vi "niRFSysCalReader Close.vi"(8 "error in":errorcluster, 11 "niRFSysCalReader Handle":T1) -> (0 "error out":errorcluster)   [LabVIEW 2016, in "niRFSysCalReader.lvlib"]
doc: "Releases the application memory created by the <b>niRFSysCalReader Initialize.vi</b>"
uses:
  niRFSysCalReader.lvlib
  _INCLUDES/niRFSysCalReader Handle.ctl
  _INCLUDES/niRFSysCalReader Core States.ctl
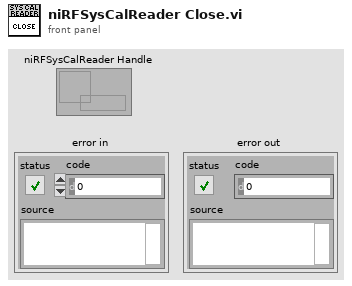
[diagram p1: front panel]
types:
  T1 = typedef "niRFSysCalReader.lvlib/niRFSysCalReader Handle.ctl" = refnum<data-value>
  T2 = typedef "niRFSysCalReader.lvlib/niRFSysCalReader Core States.ctl" = enum16{"Initialize", "Interpolator State", "Add Pathloss", "Get Pathloss", "Remove Pathloss", "Close"}
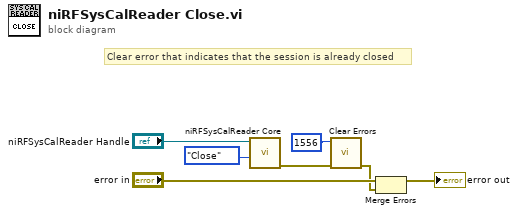
[diagram p0: block diagram]
diagram:
  # "Clear error that indicates that the session is already closed"
  n1 = call "niRFSysCalReader Core.vi"("niRFSysCalReader State"=niRFSysCalReader_Core_States."Close" ("Cal Storage"), "niRFSysCalReader Handle"="niRFSysCalReader Handle") -> ("error out"=w4:errorcluster)  [unwired: 7 in, 2 out]
  n2 = call <vilib>:"Clear Errors.vi"("error in (no error)"=w4, "specific error code to clear (0: all)"=1556) -> ("error out"=w2:errorcluster)  [unwired: 4 in, 1 out]
  n3 = Merge Errors("error in", w2) -> (→"error out":errorcluster)
